vi "Direct Motor Remote Param.vi"(0 "send cmd in":u32, 1 "ErrorString in":string, 3 "position in":i64[](array[numeric]), 4 "actual pos in":i64, 5 "remote in":bool, 7 "remote Stop in":bool, 8 "mode":T1, 9 "M-send cmd in":u32, 12 "工位数":u8, 13 "recevie cmd in":u32, 14 "index":u8, 16 "test mode in(T:manual)":bool) -> (11 "M-send cmd out":u32, 15 "recevie cmd out":u32, 17 "test mode out(T:manual)":bool, 20 "send cmd out":u32, 21 "ErrorString out":string, 23 "position out":i64[](array[numeric]), 24 "actual pos out":i64, 25 "remote out":bool, 27 "remote Stop out":bool)   [LabVIEW 2018]
uses:
  Direct Control Test/type def/Direct Value Mode.ctl
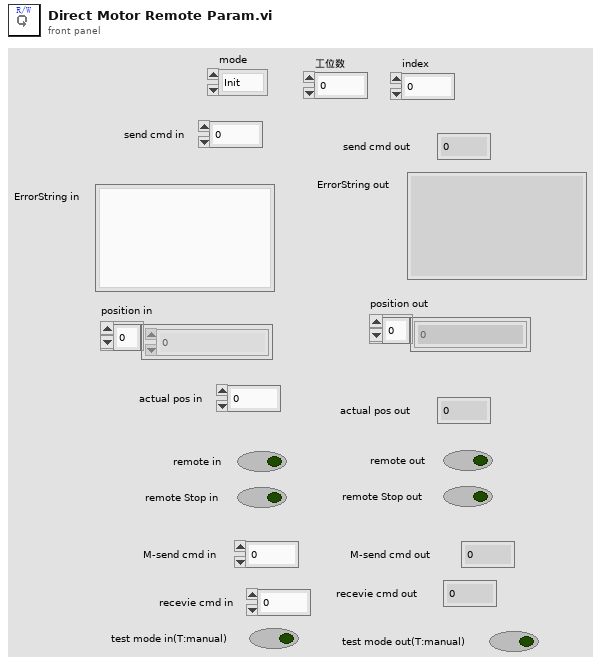
[diagram p1: front panel]
types:
  T1 = typedef "Direct Value Mode.ctl" = enum16{"Init", "read", "write send cmd", "write ER", "write position", "write AP", "write remote", "write RS", "write all input", "write Msend cmd", "write recevie cmd", "write test mode"}
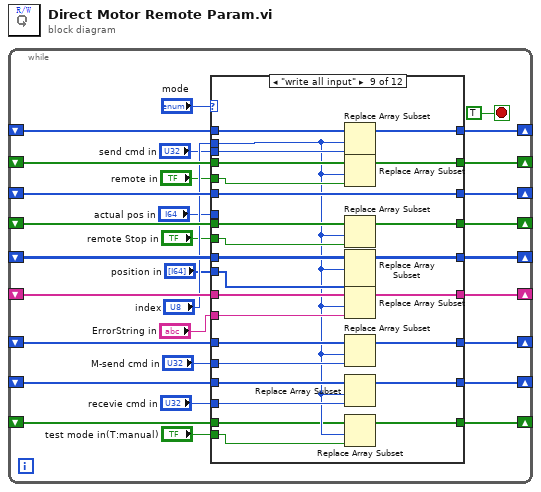
[diagram p0: block diagram]
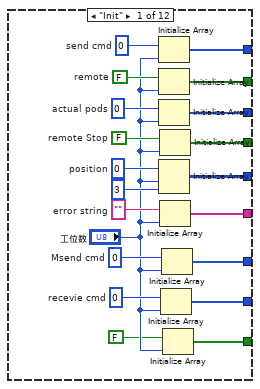
[diagram p2: hidden frame]
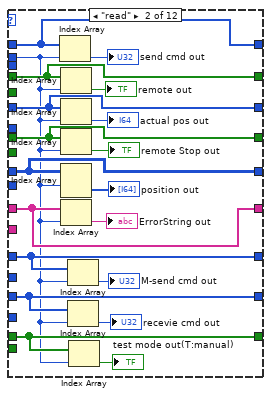
[diagram p3: hidden frame]
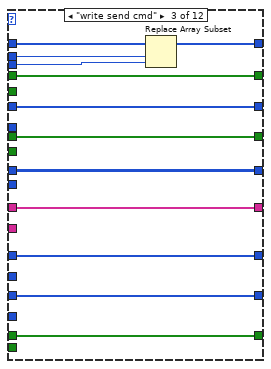
[diagram p4: hidden frame]
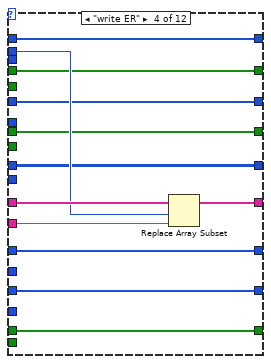
[diagram p5: hidden frame]
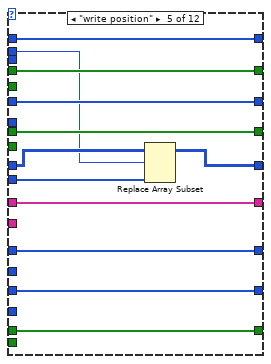
[diagram p6: hidden frame]
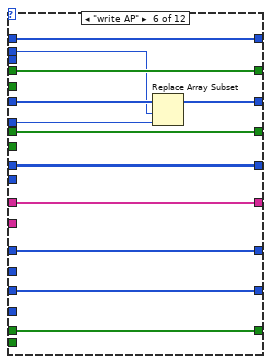
[diagram p7: hidden frame]
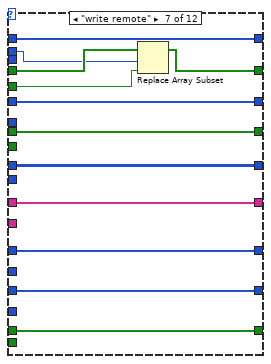
[diagram p8: hidden frame]
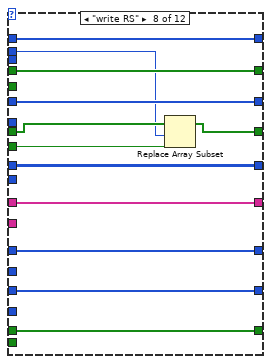
[diagram p9: hidden frame]
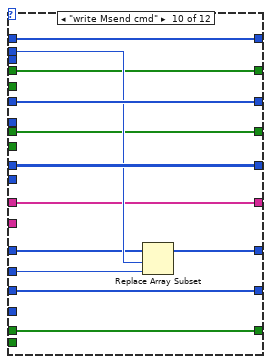
[diagram p10: hidden frame]
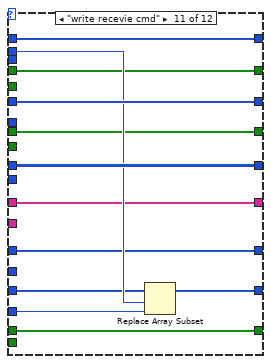
[diagram p11: hidden frame]
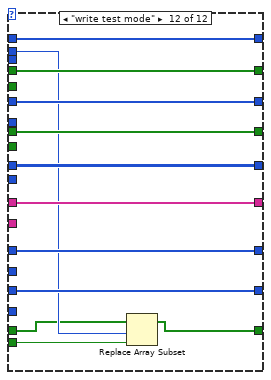
[diagram p12: hidden frame]
diagram:
  n1 = while {
    shift-right: [w29] -> _
    shift-left: _ -> [w27]
    shift-right: [w28] -> _
    shift-left: _ -> [w26]
    shift-right: [w24] -> _
    shift-left: _ -> [w23]
    shift-right: [w22] -> _
    shift-left: _ -> [w19]
    shift-right: [w21] -> _
    shift-left: _ -> [w18]
    shift-right: [w20] -> _
    shift-left: _ -> [w17]
    shift-right: [w9] -> _
    shift-left: _ -> [w7]
    shift-right: [w8] -> _
    shift-left: _ -> [w5]
    shift-right: [w1] -> _
    shift-left: _ -> [w2]
    stop <- TRUE stop-if-true
    n2 = case shown="\"write all input\"" "mode" {
      tunnel: [w49 w69 w74 w93 w105 w117 w129 w137 w166 w169 w185 w203] -> w29
      tunnel: [w48 w60 w81 w86 w104 w116 w122 w138 w164 w170 w186 w202] -> w28
      tunnel: w27 -> [_ w69 w76 w93 w105 w117 w129 w137 w167 w169 w185 w203]
      tunnel: w26 -> [_ w60 w81 w86 w104 w116 w124 w138 w165 w170 w186 w202]
      tunnel: [w46 w59 w80 w87 w103 w110 w128 w139 w155 w179 w191 w201] -> w24
      tunnel: w23 -> [_ w59 w80 w87 w103 w112 w128 w139 w155 w179 w191 w201]
      tunnel: [w43 w58 w79 w88 w102 w115 w127 w134 w162 w171 w187 w200] -> w22
      tunnel: [w40 w61 w78 w89 w98 w114 w126 w140 w146 w178 w190 w199] -> w21
      tunnel: [w38 w62 w77 w90 w101 w113 w125 w141 w160 w172 w188 w197] -> w20
      tunnel: w19 -> [_ w58 w79 w88 w102 w115 w127 w136 w163 w171 w187 w200]
      tunnel: w18 -> [_ w61 w78 w89 w100 w114 w126 w140 w148 w178 w190 w199]
      tunnel: w17 -> [_ w62 w77 w92 w101 w113 w125 w141 w161 w172 w188 w197]
      tunnel: "index" -> [_ w52 w75 w91 w99 w111 w123 w135 w145 w177 w189 w195]
      tunnel: "remote Stop in" -> [_ _ _ _ _ _ _ w133 w157 _ _ _]
      tunnel: "remote in" -> [_ _ _ _ _ _ w121 _ w158 _ _ _]
      tunnel: "actual pos in" -> [_ _ _ _ _ w109 _ _ _ _ _ _]
      tunnel: "position in" -> [_ _ _ _ w97 _ _ _ w147 _ _ _]
      tunnel: "ErrorString in" -> [_ _ _ w85 _ _ _ _ w156 _ _ _]
      tunnel: "send cmd in" -> [_ _ w73 _ _ _ _ _ w159 _ _ _]
      tunnel: [w36 w57 w72 w84 w96 w108 w120 w132 w152 w174 w184 w198] -> w9
      tunnel: [w34 w55 w71 w83 w95 w107 w119 w131 w149 w173 w182 w196] -> w8
      tunnel: w7 -> [_ w57 w72 w84 w96 w108 w120 w132 w154 w176 w184 w198]
      tunnel: "M-send cmd in" -> [_ _ _ _ _ _ _ _ w153 w175 _ _]
      tunnel: w5 -> [_ w55 w71 w83 w95 w107 w119 w131 w151 w173 w183 w196]
      tunnel: "recevie cmd in" -> [_ _ _ _ _ _ _ _ w150 _ w181 _]
      tunnel: "test mode in(T:manual)" -> [_ _ _ _ _ _ _ _ w143 _ _ w194]
      tunnel: w2 -> [_ w53 w70 w82 w94 w106 w118 w130 w144 w168 w180 w192]
      tunnel: [w31 w53 w70 w82 w94 w106 w118 w130 w142 w168 w180 w193] -> w1
      frame "Init" {
        w35 = i64 0  # recevie cmd
        w37 = i64 0  # Msend cmd
        w39 = ""  # error string
        w41 = i16 0  # position
        w44 = FALSE  # remote Stop
        w47 = i64 0  # actual pods
        w45 = FALSE  # remote
        w50 = i64 0  # send cmd
        n3 = Initialize Array(w50, "工位数") -> (w49:i64[])
        n4 = Initialize Array(w45, "工位数") -> (w48:bool[])
        n5 = Initialize Array(w47, "工位数") -> (w46:i64[])
        n6 = Initialize Array(w41, "工位数", 3 ("维数大小")) -> (w40:i16[][])
        n7 = Initialize Array(w44, "工位数") -> (w43:bool[])
        n8 = Initialize Array(w39, "工位数") -> (w38:string[])
        n9 = Initialize Array(w35, "工位数") -> (w34:i64[])
        n10 = Initialize Array(w37, "工位数") -> (w36:i64[])
        n11 = Initialize Array(FALSE, "工位数") -> (w31:bool[])
      }
      frame "read" {
        n12 = Index Array(array=w69, index=w52) -> (element=→"send cmd out":i64)
        n13 = Index Array(array=w60, index=w52) -> (element=→"remote out":bool)
        n14 = Index Array(array=w59, index=w52) -> (element=→"actual pos out":i64)
        n15 = Index Array(array=w58, index=w52) -> (element=→"remote Stop out":bool)
        n16 = Index Array(array=w61, index (row)=w52) -> (element=→"position out":i16[])  [unwired: 1 in]
        n17 = Index Array(array=w62, index=w52) -> (element=→"ErrorString out":string)
        n18 = Index Array(array=w57, index=w52) -> (element=→"M-send cmd out":i64)
        n19 = Index Array(array=w55, index=w52) -> (element=→"recevie cmd out":i64)
        n20 = Index Array(array=w53, index=w52) -> (element=→"test mode out(T:manual)":bool)
      }
      frame "write send cmd" {
        n21 = Replace Array Subset(array=w76, new element=w73, index=w75) -> (w74:i64[])
      }
      frame "write ER" {
        n22 = Replace Array Subset(array=w92, new element=w85, index=w91) -> (w90:string[])
      }
      frame "write position" {
        n23 = Replace Array Subset(array=w100, new element=w97, index (row)=w99) -> (w98:i16[][])  [unwired: 1 in]
      }
      frame "write AP" {
        n24 = Replace Array Subset(array=w112, new element=w109, index=w111) -> (w110:i64[])
      }
      frame "write remote" {
        n25 = Replace Array Subset(array=w124, new element=w121, index=w123) -> (w122:bool[])
      }
      frame "write RS" {
        n26 = Replace Array Subset(array=w136, new element=w133, index=w135) -> (w134:bool[])
      }
      frame "write all input" {
        n27 = Replace Array Subset(array=w167, new element=w159, index=w145) -> (w166:i64[])
        n28 = Replace Array Subset(array=w165, new element=w158, index=w145) -> (w164:bool[])
        n29 = Replace Array Subset(array=w163, new element=w157, index=w145) -> (w162:bool[])
        n30 = Replace Array Subset(array=w148, new element=w147, index (row)=w145) -> (w146:i16[][])  [unwired: 1 in]
        n31 = Replace Array Subset(array=w161, new element=w156, index=w145) -> (w160:string[])
        n32 = Replace Array Subset(array=w154, new element=w153, index=w145) -> (w152:i64[])
        n33 = Replace Array Subset(array=w151, new element=w150, index=w145) -> (w149:i64[])
        n34 = Replace Array Subset(array=w144, new element=w143, index=w145) -> (w142:bool[])
      }
      frame "write Msend cmd" {
        n35 = Replace Array Subset(array=w176, new element=w175, index=w177) -> (w174:i64[])
      }
      frame "write recevie cmd" {
        n36 = Replace Array Subset(array=w183, new element=w181, index=w189) -> (w182:i64[])
      }
      frame "write test mode" {
        n37 = Replace Array Subset(array=w192, new element=w194, index=w195) -> (w193:bool[])
      }
    }
  }
